vi "Parameters - Update.vi"(4 "Parameter (End Dwell Temp)":dbl, 5 "Variant Allowed (Summarised)":bool, 6 "Parameter (Start Dwell Temp)":dbl, 7 "Parameter (Current Dwell Temp)":dbl, 9 "Parameter (End Dwell Time)":timestamp, 10 "Parameter (Start Dwell Time)":timestamp, 11 "Info.":T2={"Ref WPS"="", "Hold. Temp."="", "Info. Temperature Units"="", "Variant Allowed (Hold Temp)"=5.0, "Info. Temperature Units 2"="", "Variant Allowed (Hold Temp)"=FALSE, "Hold. Time (hour:minute)"="00:00", "Variant Allowed (Hold Time)"=5.0, "Variant Allowed (Hold Time)"=FALSE, "WPS"=""} {"Variant Allowed (Hold Temp)" format="%.1f"}) -> (0 "Variant Allowed (Hold Time)":bool, 1 "Cluster":T1, 2 "Variant Allowed (Current Hold Temp)":bool, 3 "Parameters":string[][](array[string]))   [LabVIEW 2013]
uses:
  Controls/Execute - Info.ctl
  Controls/Global SRTRS.vi
panel:
  out "time stamp":timestamp
  out "Process Status":bool
  # "Min"
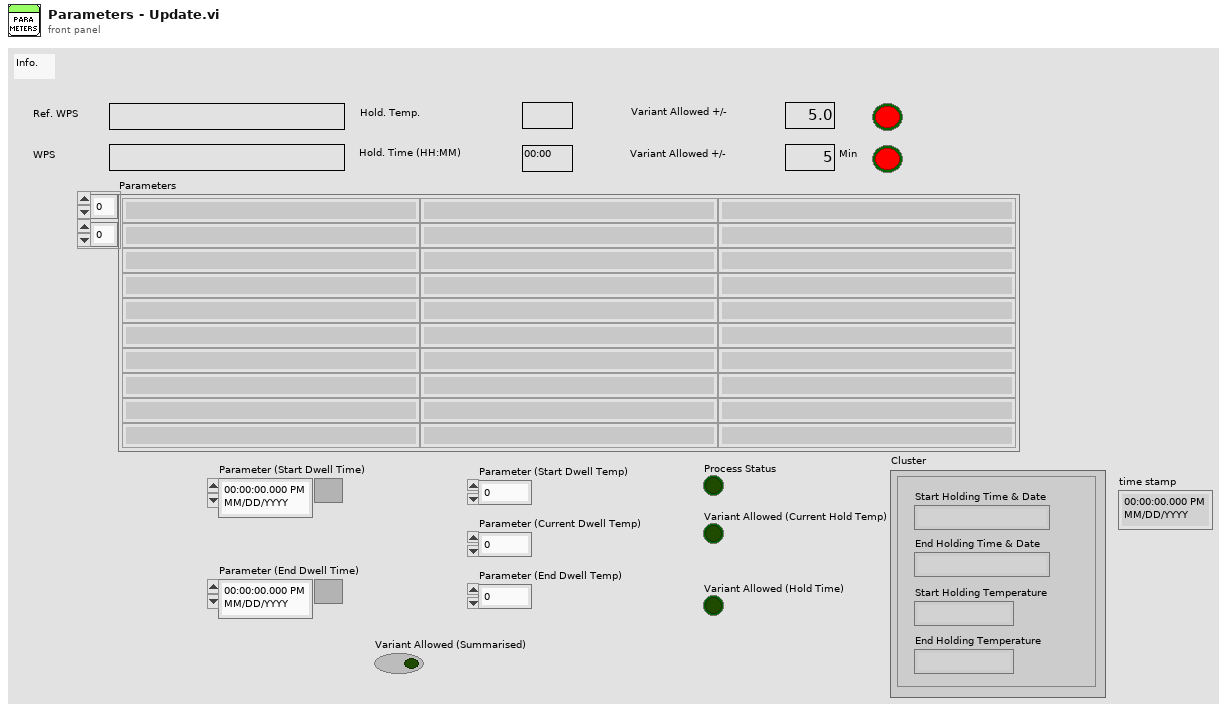
[diagram p1: front panel]
types:
  T1 = cluster{"Start Holding Time & Date":string, "End Holding Time & Date":string, "Start Holding Temperature":string, "End Holding Temperature":string}
  T2 = typedef "Execute - Info.ctl" = cluster{"Ref WPS":string, "Hold. Temp.":string, "Info. Temperature Units":string, "Variant Allowed (Hold Temp)":dbl, "Info. Temperature Units 2":string, "Variant Allowed (Hold Temp)":bool, "Hold. Time (hour:minute)":string, "Variant Allowed (Hold Time)":dbl, "Variant Allowed (Hold Time)":bool, "WPS":string}
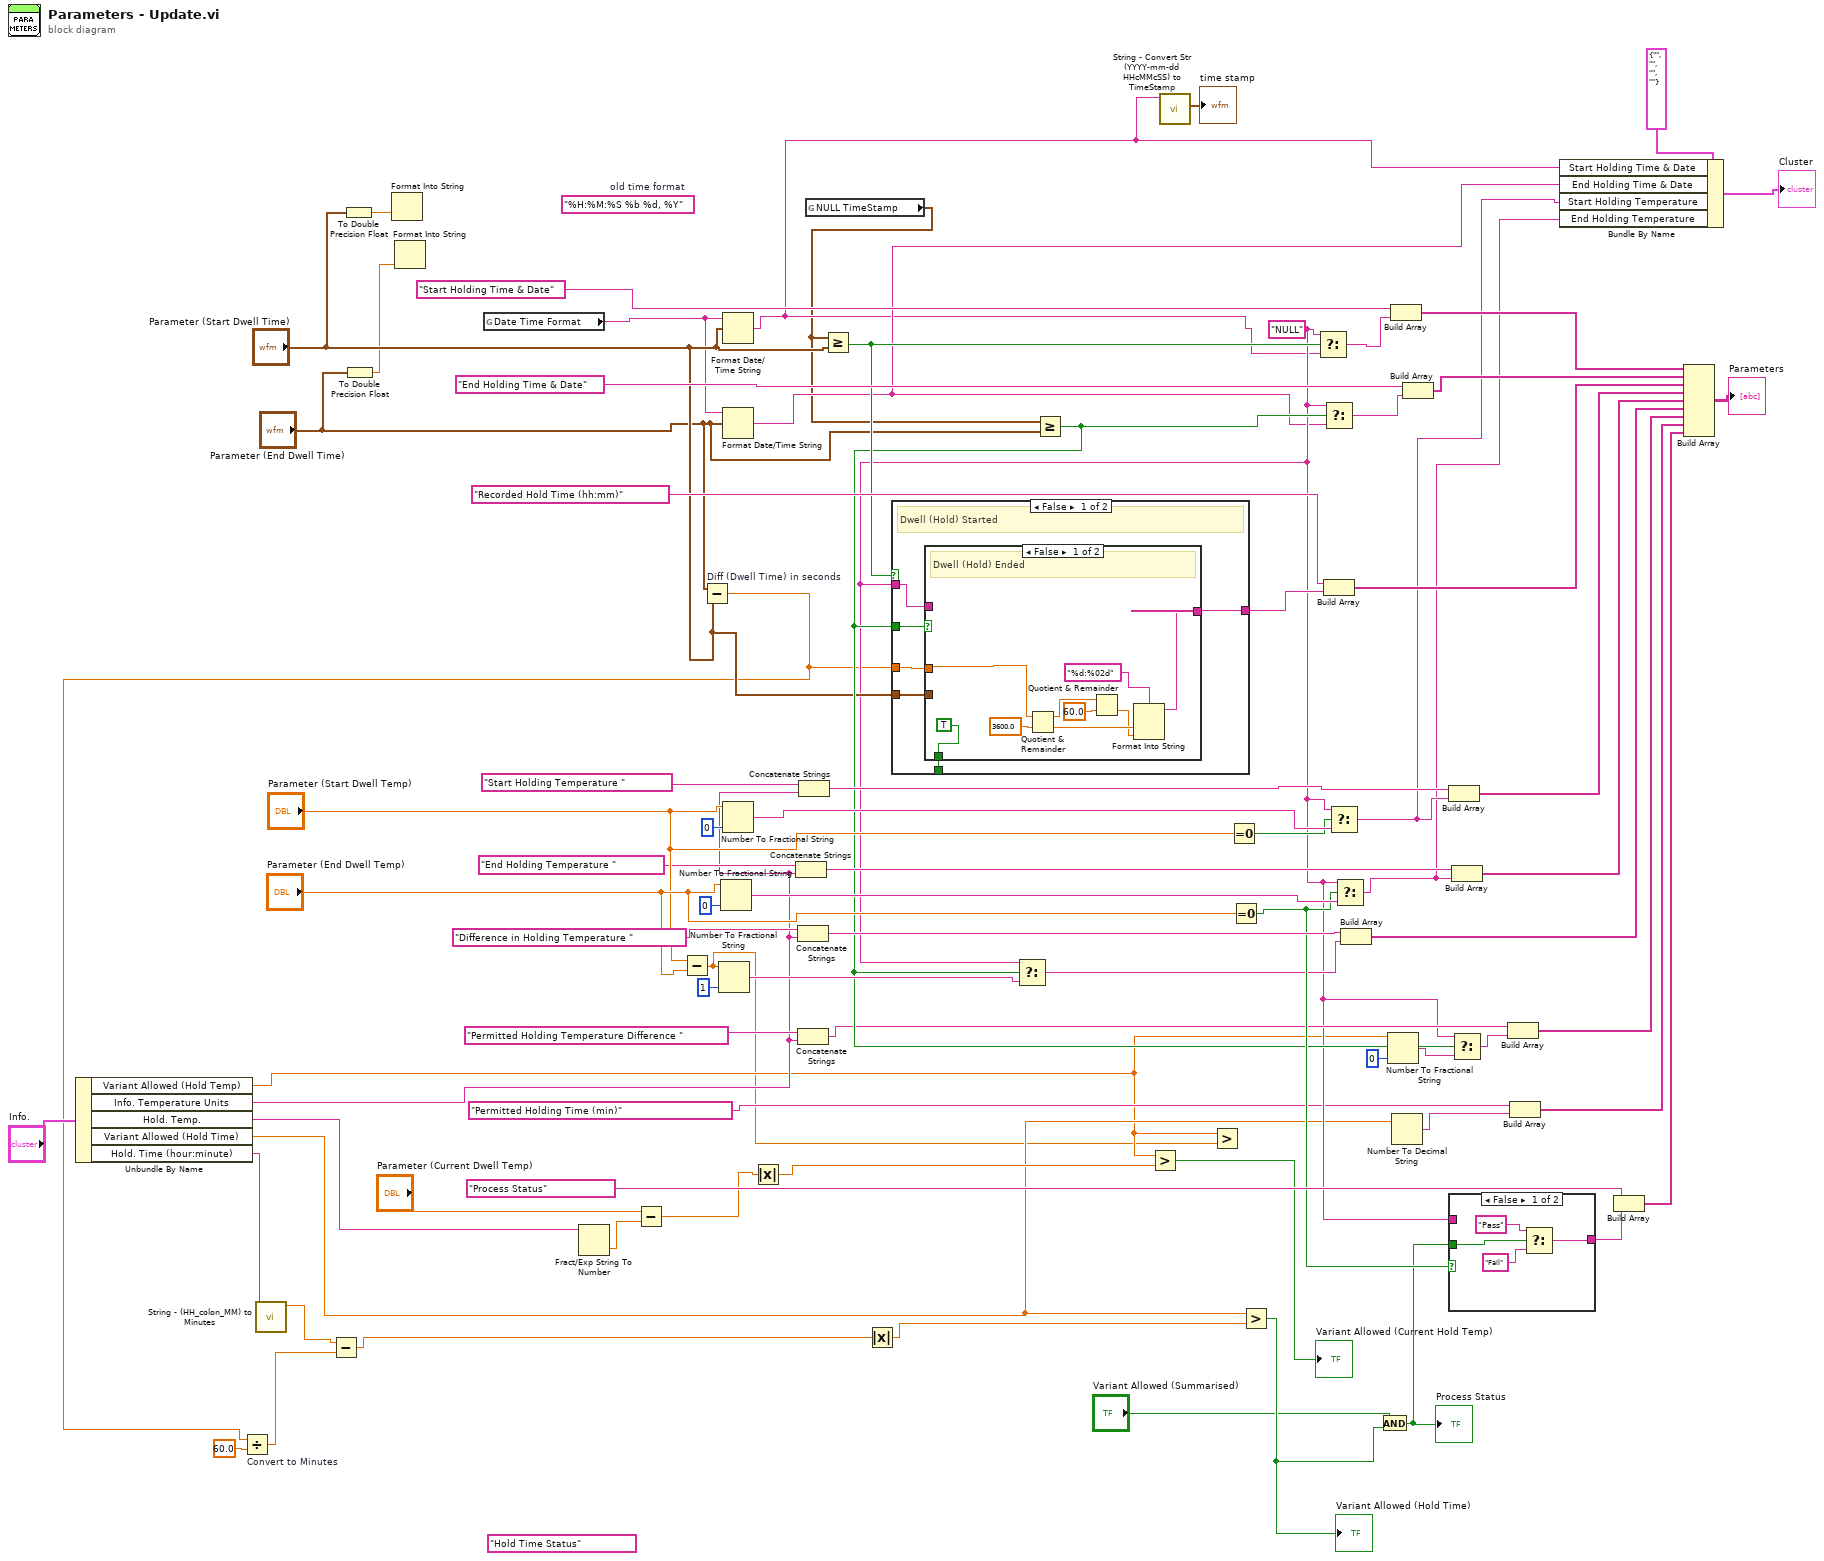
[diagram p0: block diagram]
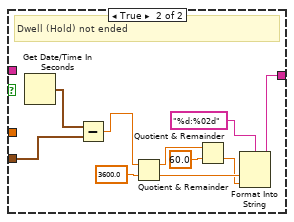
[diagram p2: hidden frame]
diagram:
  (unwired) "%H:%M:%S %b %d, %Y"  # old time format
  (unwired) "Hold Time Status"
  w27 = "NULL"
  n1 = Unbundle By Name("Info.") -> ("Variant Allowed (Hold Temp)"=w12:dbl, "Info. Temperature Units"=w15:string, "Hold. Temp."=w16:string, "Variant Allowed (Hold Time)"=w17:dbl, "Hold. Time (hour:minute)"=w4:string)
  n2 = call "String - (HH_colon_MM) to Minutes.vi"("Hold Time (HH:MM)"=w4) -> ("minutes"=w2:dbl)  [unwired: 10 in]
  n3 = To Double Precision Float(number="Parameter (Start Dwell Time)") -> (double precision float=w30:dbl)
  n4 = To Double Precision Float(number="Parameter (End Dwell Time)") -> (double precision float=w29:dbl)
  n5 = Format Into String(w30) -> ()  [unwired: 3 in, 2 out]
  n6 = Format Into String(w29) -> ()  [unwired: 3 in, 2 out]
  n7 = global read "Global SRTRS.vi" "Date Time Format"() -> (w9:string)
  n8 = Fract/Exp String To Number(string=w16) -> (number=w23:dbl)  [unwired: 3 in, 1 out]
  n9 = Subtract(x="Parameter (Current Dwell Temp)", y=w23) -> (x-y=w22:dbl)
  n10 = Subtract(x="Parameter (Start Dwell Temp)", y="Parameter (End Dwell Temp)") -> (x-y=w11:dbl)
  n11 = Subtract "Diff (Dwell Time) in seconds"(x="Parameter (End Dwell Time)", y="Parameter (Start Dwell Time)") -> (x-y=w25:dbl)
  n12 = Divide "Convert to Minutes"(x=w25, y=60.0) -> (x/y=w3:dbl)
  n13 = Subtract(x=w2, y=w3) -> (x-y=w1:dbl)
  n14 = Number To Fractional String(number=w11, precision (6)=i16 1) -> (F-format string=w44:string)  [unwired: 2 in]
  n15 = Number To Fractional String(number="Parameter (End Dwell Temp)", precision (6)=i16 0) -> (F-format string=w79:string)  [unwired: 2 in]
  n16 = Format Date/Time String(time format string (%c)=w9, seconds (now)="Parameter (Start Dwell Time)") -> (date/time string=w7:string)  [unwired: 1 in]
  n17 = Format Date/Time String(time format string (%c)=w9, seconds (now)="Parameter (End Dwell Time)") -> (date/time string=w8:string)  [unwired: 1 in]
  n18 = Number To Fractional String(number="Parameter (Start Dwell Temp)", precision (6)=i16 0) -> (F-format string=w77:string)  [unwired: 2 in]
  n19 = Absolute Value(x=w22) -> (abs(x)=w65:dbl)
  n20 = Concatenate Strings("End Holding Temperature ", w15) -> (w70:string)
  n21 = Concatenate Strings("Difference in Holding Temperature ", w15) -> (w72:string)
  n22 = Concatenate Strings("Permitted Holding Temperature Difference ", w15) -> (w41:string)
  n23 = Concatenate Strings("Start Holding Temperature ", w15) -> (w68:string)
  n24 = global read "Global SRTRS.vi" "NULL TimeStamp"() -> (w5:timestamp)
  n25 = Greater Or Equal?(x=w5, y="Parameter (Start Dwell Time)") -> (x >= y?=w46:bool)
  n26 = Absolute Value(x=w1) -> (abs(x)=w28:dbl)
  n27 = Greater Or Equal?(x=w5, y="Parameter (End Dwell Time)") -> (x >= y?=w43:bool)
  n28 = case shown="False" w46 {
    tunnel: w25 -> [w82 _]
    tunnel: w27 -> [w83 w105]
    tunnel: [w84 w105] -> w45
    tunnel: w43 -> [w85 _]
    tunnel: "Parameter (Start Dwell Time)" -> [w81 _]
    tunnel: [w80 _] -> _
    frame False {
      # "Dwell (Hold) Started"
      n29 = case shown="False" w85 {
        tunnel: [w87 w95] -> w84
        tunnel: w83 -> [_ _]
        tunnel: w82 -> [w88 _]
        tunnel: w81 -> [_ w104]
        tunnel: [TRUE _] -> w80
        frame False {
          # "Dwell (Hold) Ended"
          n30 = Quotient & Remainder(x=w88, y=3600.0) -> (x-y*floor(x/y)=w89:dbl, floor(x/y)=w92:dbl)
          n31 = Quotient & Remainder(x=w89, y=60.0) -> (floor(x/y)=w90:dbl)  [unwired: 1 out]
          n32 = Format Into String(format string="%d:%02d", w92, w90) -> (resulting string=w87:string)  [unwired: 2 in, 1 out]
        }
        frame True {
          # "Dwell (Hold) not ended"
          n33 = Get Date/Time In Seconds() -> (seconds since 1Jan1904=w103:timestamp)
          n34 = Subtract(x=w103, y=w104) -> (x-y=w96:dbl)
          n35 = Quotient & Remainder(x=w96, y=3600.0) -> (x-y*floor(x/y)=w97:dbl, floor(x/y)=w100:dbl)
          n36 = Quotient & Remainder(x=w97, y=60.0) -> (floor(x/y)=w98:dbl)  [unwired: 1 out]
          n37 = Format Into String(format string="%d:%02d", w100, w98) -> (resulting string=w95:string)  [unwired: 2 in, 1 out]
        }
      }
    }
    frame True {
      # "Dwell (Hold) not started"
    }
  }
  n38 = Select(t=w27, s=w43, f=w44) -> (s? t:f=w42:string)
  n39 = Greater?(x=w12, y=w65) -> (0:→"Variant Allowed (Current Hold Temp)":bool)
  n40 = call "String - Convert Str (YYYY-mm-dd HHcMMcSS) to TimeStamp.vi"("YYYY-mm-dd HH:MM:SS (String)"=w7) -> ("time stamp"=→"time stamp":timestamp)  [unwired: 9 in, 1 out]
  n41 = Greater?(x=w12, y=w11) -> ()  [unwired: 1 out]
  n42 = Equal To 0?(x="Parameter (Start Dwell Temp)") -> (x = 0?=w76:bool)
  n43 = Equal To 0?(x="Parameter (End Dwell Temp)") -> (x = 0?=w47:bool)
  n44 = Greater?(x=w17, y=w28) -> (0:w20:bool)
  "Variant Allowed (Hold Time)" <- w20
  n45 = Select(t=w27, s=w46, f=w7) -> (s? t:f=w36:string)
  n46 = Select(t=w27, s=w43, f=w8) -> (s? t:f=w35:string)
  n47 = Build Array("Recorded Hold Time (hh:mm)", w45) -> (w57:string[])
  n48 = Select(t=w27, s=w76, f=w77) -> (s? t:f=w34:string)
  n49 = Select(t=w27, s=w47, f=w79) -> (s? t:f=w33:string)
  n50 = Build Array(w72, w42) -> (w73:string[])
  n51 = And(x="Variant Allowed (Summarised)", y=w20) -> (x .and. y?=w14:bool)
  "Process Status" <- w14
  n52 = Number To Fractional String(number=w12, precision (6)=i16 0) -> (F-format string=w40:string)  [unwired: 2 in]
  n53 = Build Array("Start Holding Time & Date", w36) -> (w56:string[])
  n54 = Number To Decimal String(number=w17) -> (decimal integer string=w18:string)  [unwired: 1 in]
  n55 = Build Array("End Holding Time & Date", w35) -> (w61:string[])
  n56 = Build Array(w68, w34) -> (w69:string[])
  n57 = case shown="False" w47 {
    tunnel: [w109 w110] -> w67
    tunnel: w14 -> [w108 _]
    tunnel: w27 -> [_ w110]
    frame False {
      n58 = Select(t="Pass" ("element"), s=w108, f="Fail" ("element")) -> (s? t:f=w109:string)
    }
    frame True {
    }
  }
  n59 = Build Array(w70, w33) -> (w71:string[])
  n60 = Select(t=w27, s=w43, f=w40) -> (s? t:f=w39:string)
  n61 = Build Array(w41, w39) -> (w58:string[])
  n62 = Build Array("Permitted Holding Time (min)", w18) -> (w13:string[])
  n63 = Bundle By Name(cluster=T1 {"Start Holding Time & Date"="", "End Holding Time & Date"="", "Start Holding Temperature"="", "End Holding Temperature"=""} ("Cluster"), "Start Holding Time & Date"=w7, "End Holding Time & Date"=w8, "Start Holding Temperature"=w34, "End Holding Temperature"=w33) -> (→"Cluster":T1)
  n64 = Build Array("Process Status", w67) -> (w59:string[])
  n65 = Build Array(w56, w61, w57, w69, w71, w73, w58, w13, w59) -> (→"Parameters":string[][])
